vi "Counter - Single Pulse Output.vi"() -> ()   [LabVIEW 2022 SP3]
doc: "This example demonstrates how to generate a single pulse using a counter output. \n\nThe single pulse may be triggered once or repeatedly from an external source."
uses:
  <vilib>/Utility/error.llb/DialogType.ctl
  <vilib>/DAQmx/create/channels.llb/DAQmx Create Channel (CO-Pulse Generation-Time).vi
  <vilib>/DAQmx/configure/trigger.llb/DAQmx Start Trigger (Digital Edge).vi
  <resource>/objmgr/daqmx.rc
panel:
  in  "Pulse Duration":dbl=1.0 format="%.6f"
  in  "Output Terminal":tag="/Dev1/PFI12"
  in  "Trigger Type":enum32{"No Trigger", "Digital Start"}(tab)
  in  "Retriggerable":bool
  in  "Edge":i32(ring)=10280 items=["Rising"=10280, "Falling"=10171]
  in  "Digital Trigger Source":tag
  in  "Stop":bool
  in  "Counter":tag="Dev1/ctr0"
  # "Channel Settings"
  # "Trigger Settings"
  # "To configure and use a trigger you must have the necessary tab selected above."
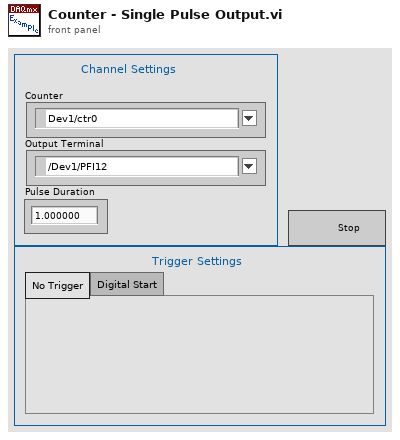
[diagram p1: front panel]
types:
  T1 = typedef "DialogType.ctl" = u16
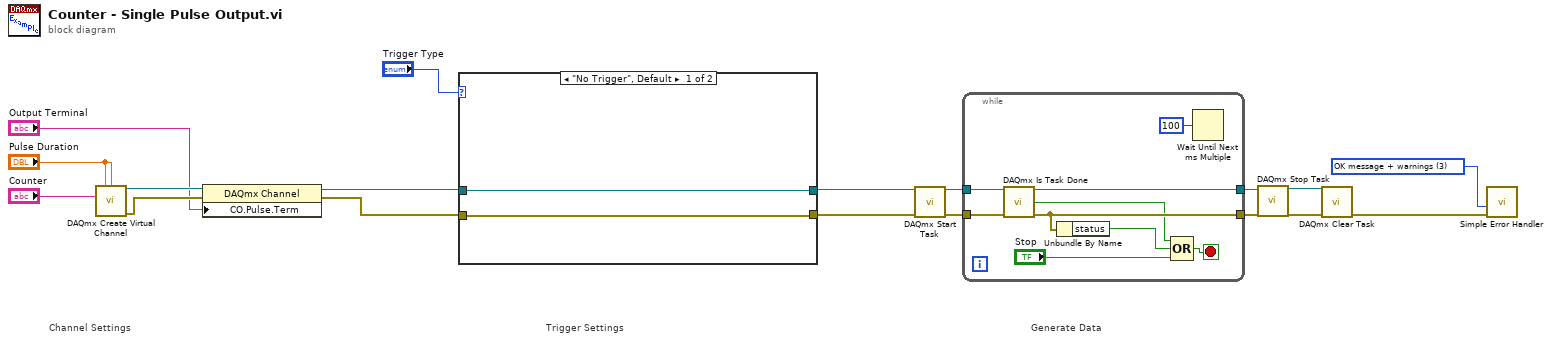
[diagram p0: block diagram]
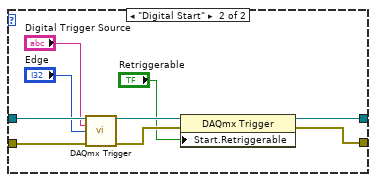
[diagram p2: hidden frame]
diagram:
  w1 = T1 3 items=["no dialog", "OK message", "continue or stop message", "OK message + warnings", "continue/stop + warnings"] ("type of dialog (OK msg:1)")
  # "Generate Data"
  # "Trigger Settings"
  # "Channel Settings"
  n1 = call-poly <vilib>:"DAQmx Create Virtual Channel.vi"("high time"="Pulse Duration", "low time"="Pulse Duration", "counter"="Counter") -> ("task out"=w11:refnum<k21>, "error out"=w10:errorcluster)  [unwired: 11 in]
  n2 = property class="DAQmx Channel"(reference=w11, error in=w10, "CO.Pulse.Term"="Output Terminal") -> (reference out=w7:refnum<k21>, error out=w8:errorcluster)
  n3 = case shown="\"No Trigger\", Default" "Trigger Type" {
    tunnel: w7 -> [w20 w29]
    tunnel: w8 -> [w19 w28]
    tunnel: [w20 w25] -> w12
    tunnel: [w19 w24] -> w13
    frame "No Trigger", Default {
    }
    frame "Digital Start" {
      n4 = call-poly <vilib>:"DAQmx Trigger.vi"("task/channels in"=w29, "source"="Digital Trigger Source", "edge"="Edge", "error in"=w28) -> ("task out"=w22:refnum<k21>, "error out"=w23:errorcluster)  [unwired: 10 in]
      n5 = property class="DAQmx Trigger"(reference=w22, error in=w23, "Start.Retriggerable"="Retriggerable") -> (reference out=w25:refnum<k21>, error out=w24:errorcluster)
    }
  }
  n6 = call <vilib>:"DAQmx Start Task.vi"("task/channels in"=w12, "error in"=w13) -> ("task out"=w18:refnum<k21>, "error out"=w17:errorcluster)  [unwired: 12 in]
  n7 = while {
    tunnel: w18 -> [w38]
    tunnel: w17 -> [w37]
    tunnel: [w34] -> w4
    tunnel: [w35] -> w5
    stop <- w36 stop-if-true
    n8 = call <vilib>:"DAQmx Is Task Done.vi"("task/channels in"=w38, "error in"=w37) -> ("task out"=w35:refnum<k21>, "task done?"=w30:bool, "error out"=w34:errorcluster)  [unwired: 11 in]
    n9 = Unbundle By Name(w34) -> ("status"=w33:bool)
    n10 = Compound Arithmetic op=OR(w30, w33, "Stop") -> (w36:bool)
    n11 = Wait Until Next ms Multiple(millisecond multiple=u32 100) -> ()  [unwired: 1 out]
  }
  n12 = call <vilib>:"DAQmx Stop Task.vi"("task/channels in"=w5, "error in"=w4) -> ("task out"=w3:refnum<k21>, "error out"=w2:errorcluster)  [unwired: 12 in]
  n13 = call <vilib>:"DAQmx Clear Task.vi"("task in"=w3, "error in"=w2) -> ("error out"=w16:errorcluster)  [unwired: 13 in]
  n14 = call <vilib>:"Simple Error Handler.vi"("type of dialog (OK msg:1)"=w1, "error in (no error)"=w16) -> ()  [unwired: 3 in, 5 out]
